vi "Driver Server.vi"() -> ()   [LabVIEW 2010]
uses:
  <vilib>/Instr/_visa.llb/VISA Configure Serial Port (Instr).vi
panel:
  in  "Stop":bool
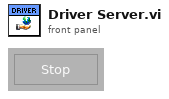
[diagram p1: front panel]
types:
  T1 = enum32{"invalid app kind", "Development System", "Run Time System", "Student Edition", "Embedded LabVIEW", "Evaluation", "Custom"}
  T2 = typedef "Path InitPaths__FS.ctl" = cluster{"Ctrller CFG":path, "INI":path, "Profile":path, "EventLog":path, "Data":path}
  T3 = typedef "Controller Configuration__CHC.ctl" = cluster{"Ctrller Type":T4, "Ctrller Name":string, "Ctrller Addr":string, "Server IP":string, "Conn Result":string, "Port":string, "Baud":dbl}
  T4 = typedef "Controller Configuration__Ctrller Type.ctl" = enum16{"F4S/D", "Synergy"}
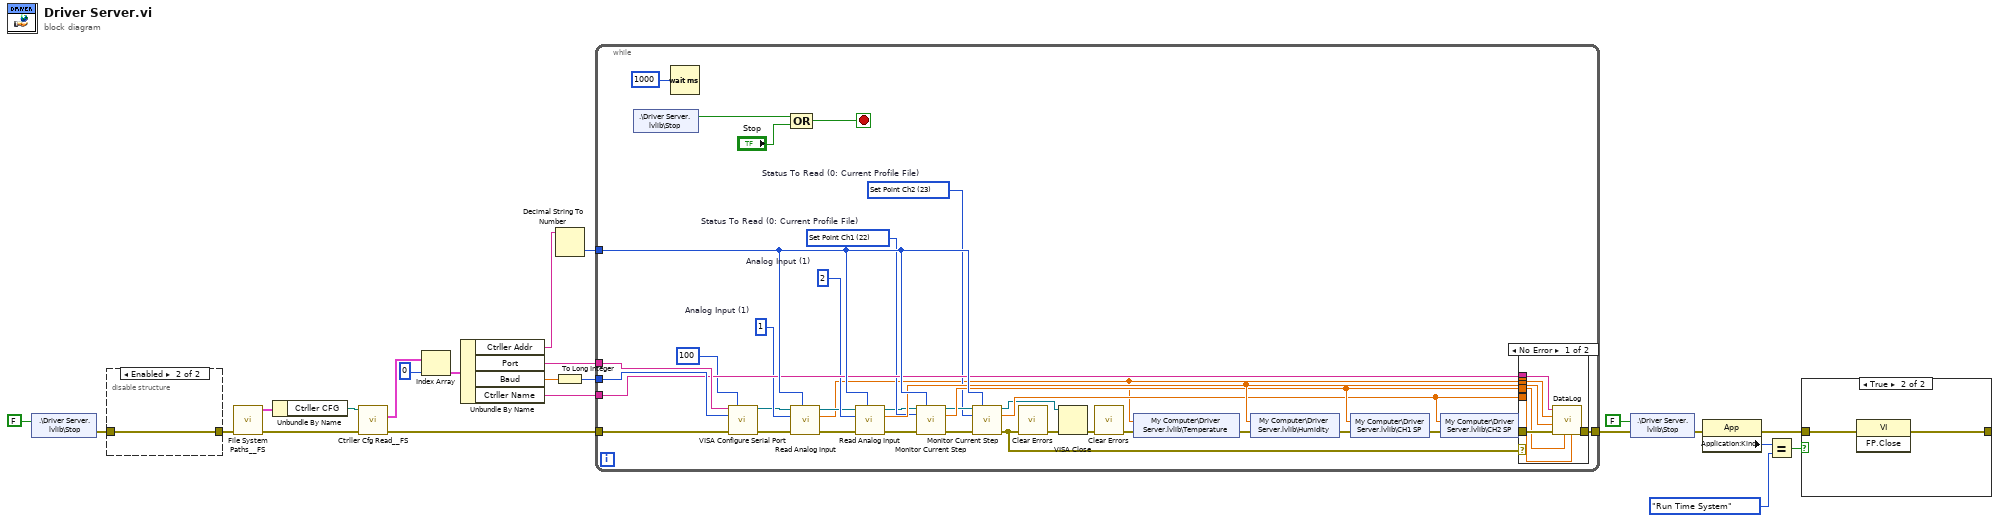
[diagram p0: block diagram]
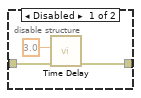
[diagram p3: hidden frame]
diagram:
  n1 = shared-variable ".\\Driver Server.lvlib\\Stop"(FALSE ("Stop")) -> (error out=w10:errorcluster)  [unwired: 1 in]
  n2 = disable-structure shown="Enabled" {
    disable-tunnel: w10 -> [w25 w27]
    disable-tunnel: [w24 w27] -> w9
    frame Disabled {
      n3 = call "Time Delay"("error in (no error)"=w25, "Delay Time (s)"=3.0) -> ("error out"=w24:errorcluster)  [unwired: 9 in]
    }
    frame Enabled {
    }
  }
  n4 = call "File System Paths__FS.vi"("error in (no error)"=w9) -> ("error out"=w11:errorcluster, "FilePaths"=w22:T2)  [unwired: 8 in, 1 out]
  n5 = Unbundle By Name(w22) -> ("Ctrller CFG"=w23:path)
  n6 = call "Ctrller Cfg Read__FS.vi"("error in (no error)"=w11, "Path In"=w23) -> ("error out"=w8:errorcluster, "Ctrllers"=w21:T3[])  [unwired: 7 in, 1 out]
  n7 = Index Array(array=w21, index=0) -> (element=w19:T3)
  n8 = Unbundle By Name(w19) -> ("Ctrller Addr"=w17:string, "Port"=w18:string, "Baud"=w15:dbl, "Ctrller Name"=w13:string)
  n9 = To Long Integer(number=w15) -> (32bit integer=w14:i32)
  n10 = Decimal String To Number(string=w17) -> (number=w16:i32)  [unwired: 2 in, 1 out]
  n11 = while {
    tunnel: w18 -> [w62]
    tunnel: w16 -> [w63]
    tunnel: w14 -> [w61]
    tunnel: w13 -> [w59]
    tunnel: [w57] -> w2
    tunnel: w8 -> [w56]
    stop <- w53 stop-if-true
    w36 = u16 23 items=["Current Profile File Number", "Current Profile Step Number", "Current Profile Step Type", "Profile Ramp Waiting", "Profile Waiting For Event 1", "Profile Waiting For Event 2", "Profile Waiting For Event 3", "Profile Waiting For Event 4", "Profile Waiting Analog Input 1", "Profile Waiting Analog Input 2", "Profile Waiting Analog Input 3", "Digital Output 1", "Digital Output 2", "Digital Output 3", "Digital Output 4", "Digital Output 5", "Digital Output 6", "Digital Output 7", "Digital Output 8", "Hours Remaining", "Minutes Remaining", "Seconds Remaining", "Set Point Ch1", "Set Point Ch2", "Ch1 PID Set", "Ch2 PID Set", "Last Jump Count", "Last Jump File", "Jump Step", "End Setpoint Ch1", "End Setpoint Ch2"]  # Status To Read (0: Current Profile File)
    w35 = u16 22 items=["Current Profile File Number", "Current Profile Step Number", "Current Profile Step Type", "Profile Ramp Waiting", "Profile Waiting For Event 1", "Profile Waiting For Event 2", "Profile Waiting For Event 3", "Profile Waiting For Event 4", "Profile Waiting Analog Input 1", "Profile Waiting Analog Input 2", "Profile Waiting Analog Input 3", "Digital Output 1", "Digital Output 2", "Digital Output 3", "Digital Output 4", "Digital Output 5", "Digital Output 6", "Digital Output 7", "Digital Output 8", "Hours Remaining", "Minutes Remaining", "Seconds Remaining", "Set Point Ch1", "Set Point Ch2", "Ch1 PID Set", "Ch2 PID Set", "Last Jump Count", "Last Jump File", "Jump Step", "End Setpoint Ch1", "End Setpoint Ch2"]  # Status To Read (0: Current Profile File)
    w42 = i16 2  # Analog Input (1)
    w46 = i16 1  # Analog Input (1)
    n12 = shared-variable ".\\Driver Server.lvlib\\Stop"() -> (w54:bool)  [unwired: 1 in, 1 out]
    n13 = Wait (ms)(milliseconds to wait=u32 1000) -> ()  [unwired: 1 out]
    n14 = call-poly "VISA Configure Serial Port"("VISA resource name"=w62, "timeout (10sec)"=u32 100, "baud rate (9600)"=w61, "error in (no error)"=w56) -> ("VISA resource name out"=w45:refnum<visa-resource-name>, "error out"=w43:errorcluster)  [unwired: 10 in]
    n15 = Compound Arithmetic op=OR(w54, "Stop") -> (w53:bool)
    n16 = call "Read Analog Input.vi"("Unit Address (1)"=w63, "error in (no error)"=w43, "Analog Input (1)"=w46, "VISA resource name"=w45) -> ("error out"=w44:errorcluster, "Value"=w29:dbl, "VISA resource name out"=w41:refnum<visa-resource-name>)  [unwired: 5 in]
    n17 = call "Read Analog Input.vi"("Unit Address (1)"=w63, "error in (no error)"=w44, "Analog Input (1)"=w42, "VISA resource name"=w41) -> ("error out"=w32:errorcluster, "Value"=w58:dbl, "VISA resource name out"=w34:refnum<visa-resource-name>)  [unwired: 5 in]
    n18 = call "Monitor Current Step.vi"("VISA resource name"=w34, "Unit Address (1)"=w63, "Status To Read (0: Current Profile File)"=w35, "error in (no error)"=w32) -> ("VISA resource name out"=w37:refnum<visa-resource-name>, "Value"=w48:dbl, "error out"=w38:errorcluster)  [unwired: 9 in]
    n19 = call "Monitor Current Step.vi"("VISA resource name"=w37, "Unit Address (1)"=w63, "Status To Read (0: Current Profile File)"=w36, "error in (no error)"=w38) -> ("VISA resource name out"=w33:refnum<visa-resource-name>, "Value"=w47:dbl, "error out"=w28:errorcluster)  [unwired: 9 in]
    n20 = call <vilib>:"Clear Errors.vi"("error in (no error)"=w28) -> ("error out"=w39:errorcluster)  [unwired: 6 in]
    n21 = VISA Close(VISA resource name=w33, error in (no error)=w39) -> (error out=w31:errorcluster)
    n22 = call <vilib>:"Clear Errors.vi"("error in (no error)"=w31) -> ("error out"=w30:errorcluster)  [unwired: 6 in]
    n23 = shared-variable "My Computer\\Driver Server.lvlib\\Temperature"(w29, error in=w30) -> (error out=w55:errorcluster)
    n24 = shared-variable "My Computer\\Driver Server.lvlib\\Humidity"(w58, error in=w55) -> (error out=w51:errorcluster)
    n25 = shared-variable "My Computer\\Driver Server.lvlib\\CH1 SP"(w48, error in=w51) -> (error out=w50:errorcluster)
    n26 = shared-variable "My Computer\\Driver Server.lvlib\\CH2 SP"(w47, error in=w50) -> (error out=w49:errorcluster)
    n27 = case shown="No Error" w28 {
      tunnel: w59 -> [w70 _]
      tunnel: w29 -> [w69 _]
      tunnel: w58 -> [w68 _]
      tunnel: [w67 w71] -> w57
      tunnel: w49 -> [w66 w71]
      tunnel: w48 -> [w65 _]
      tunnel: w47 -> [w64 _]
      frame No Error {
        n28 = call "DataLog.vi"("CH2 SP"=w64, "CH1 SP"=w65, "error in (no error)"=w66, "CH2"=w68, "CH1"=w69, "Controller Name"=w70) -> ("error out"=w67:errorcluster)  [unwired: 5 in]
      }
      frame Error {
      }
    }
  }
  n29 = shared-variable ".\\Driver Server.lvlib\\Stop"(FALSE ("Stop"), error in=w2) -> (error out=w1:errorcluster)
  n30 = property class="App"(error in=w1) -> (error out=w7:errorcluster, "Application:Kind"=w6:T1)  [unwired: 1 in, 1 out]
  n31 = Equal?(x=w6, y=T1."Run Time System") -> (x = y?=w4:bool)
  n32 = case shown="True" w4 {
    tunnel: w7 -> [w72 w74]
    tunnel: [w72 w73] -> _
    frame False {
    }
    frame True {
      n33 = invoke class="VI" method="FP.Close"(error in=w74) -> (error out=w73:errorcluster)  [unwired: 2 in, 2 out]
    }
  }
